vi "Validar_Value_adc.vi"(10 "String":string, 11 "Val_ante_adc":dbl) -> (3 "Val_ante_adc 2":dbl)   [LabVIEW 2019, in "Multiple_uC.lvlib"]
uses:
  Multiple_uC.lvlib
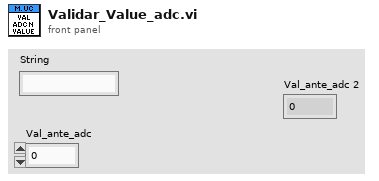
[diagram p1: front panel]
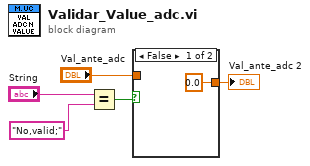
[diagram p0: block diagram]
diagram:
  n1 = Equal?(x="String", y="No,valid;") -> (x = y?=w3:bool)
  n2 = case shown="False" w3 {
    tunnel: [0.0 ("Val_ante_adc") w7] -> w1
    tunnel: "Val_ante_adc" -> [_ w7]
    frame False {
    }
    frame True {
    }
  }
  "Val_ante_adc 2" <- w1
